vi "Configure Scale.vi"(0 "VISA resource name":refnum<visa-resource-name>, 5 "Scale Per Division (1: DIV1)":i32(ring)=1 items=["DIV1"=1, "DIV2"=2, "DIV5"=5, "DIV10"=10], 9 "Vertical Scale (0: Linear)":i32(ring) items=["Linear", "Logarithmic"], 11 "error in (no error)":errorcluster) -> (4 "VISA resource name out":refnum<visa-resource-name>, 15 "error out":errorcluster)   [LabVIEW 2022 SP3, in "Agilent N934X Series.lvlib"]
doc: "Configure display scale functions of the spectrum."
uses:
  <instrlib>/Agilent N934X Series/Agilent N934X Series.lvlib
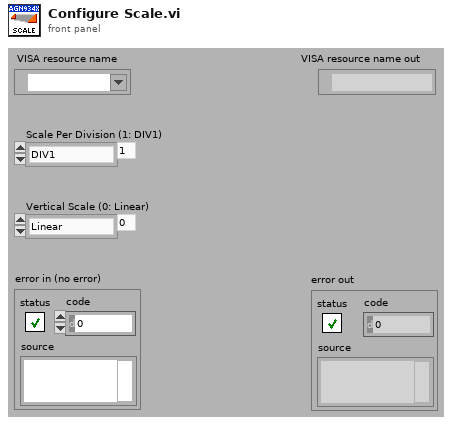
[diagram p1: front panel]
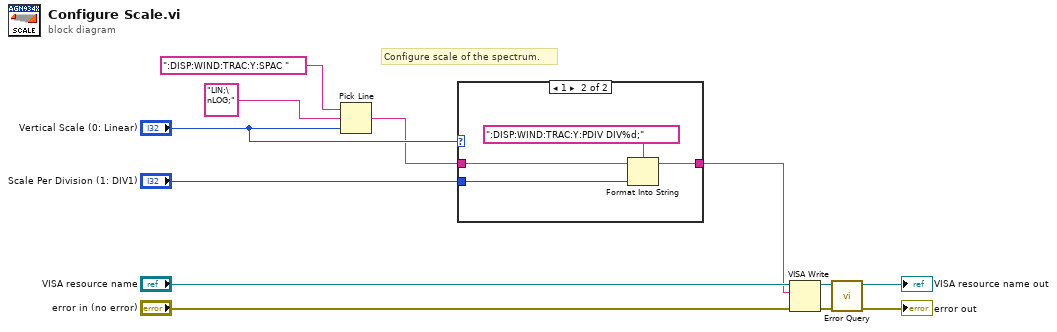
[diagram p0: block diagram]
diagram:
  # "Configure scale of the spectrum."
  n1 = Pick Line(string ("")=":DISP:WIND:TRAC:Y:SPAC ", multi-line string="LIN;\nLOG;", line index="Vertical Scale (0: Linear)") -> (output string=w2:string)
  n2 = case shown="1" "Vertical Scale (0: Linear)" {
    tunnel: w2 -> [w13 w16]
    tunnel: "Scale Per Division (1: DIV1)" -> [_ w15]
    tunnel: [w13 w14] -> w1
    frame 0, Default {
    }
    frame 1 {
      n3 = Format Into String(format string=":DISP:WIND:TRAC:Y:PDIV DIV%d;", initial string=w16, w15) -> (resulting string=w14:string)  [unwired: 1 in, 1 out]
    }
  }
  n4 = VISA Write(VISA resource name="VISA resource name", write buffer=w1, error in (no error)="error in (no error)") -> (VISA resource name out=w12:refnum<visa-resource-name>, error out=w11:errorcluster)  [unwired: 1 out]
  n5 = call <instrlib>:"Error Query.vi"("error in (no error)"=w11, "VISA resource name"=w12) -> ("error out"=→"error out":errorcluster, "VISA resource name out"=→"VISA resource name out":refnum<visa-resource-name>)  [unwired: 6 in, 2 out]
